vi "Build Header Frame.vi"(8 "error in (no error)":errorcluster, 9 "system info in":refnum<class "PMU System Info.lvclass">) -> (0 "error out":errorcluster, 1 "system info out":refnum<class "PMU System Info.lvclass">, 3 "header frame":string)   [LabVIEW 2013, in "NI_EP_PMU.lvlib"]
doc: "Builds a header frame as defined in IEEE Std C37.118.2-2011."
uses:
  <vilib>/addons/Electrical Power/PMU/NI_EP_PMU.lvlib
  <vilib>/addons/Electrical Power/PMU/Common/Classes/PMU System Info/PMU System Info.lvclass
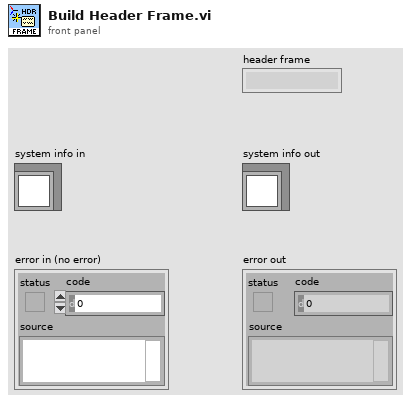
[diagram p1: front panel]
types:
  T1 = typedef "NI_EP_PMU.lvlib/pmu_CFG for Data Frame.ctl" = enum8{"CFG-2", "CFG-3"}
  T2 = typedef "NI_EP_PMU.lvlib/pmu_CFG Class.ctl" = cluster{"station name":string, "PMU ID":u16, "time base":u32, "nominal frequency":enum16{"50 Hz", "60 Hz"}, "reporting rate":i16, "phasor number":u16, "analog number":u16, "digital number":u16, "channel names":string[], "phasor units":u32[], "analog units":u32[], "digital units":u32[], "data format":u16, "number of PMUs":u16}
  T3 = typedef "NI_EP_PMU.lvlib/pmu_CFG-3 Class.ctl" = cluster{"station name":string, "PMU ID":u16, "global PMU ID":u64, "time base":u32, "nominal frequency":enum16{"50 Hz", "60 Hz"}, "reporting rate":i16, "phasor number":u16, "analog number":u16, "digital number":u16, "channel names":string[], "phasor scale first 4 bytes":u32[], "phasor scale factors":sgl[], "phasor angle offsets [rad]":sgl[], "analog scale factors":sgl[], "analog magnitude offsets":sgl[], "digital units":u32[], "data format":u16, "number of PMUs":u16}
  T4 = typedef "LVDateTimeRec.ctl" = cluster{"fractional second":dbl, "second":i32, "minute":i32, "hour":i32, "day of month":i32, "month":i32, "year":i32, "day of week":i32, "day of year":i32, "DST":i32}
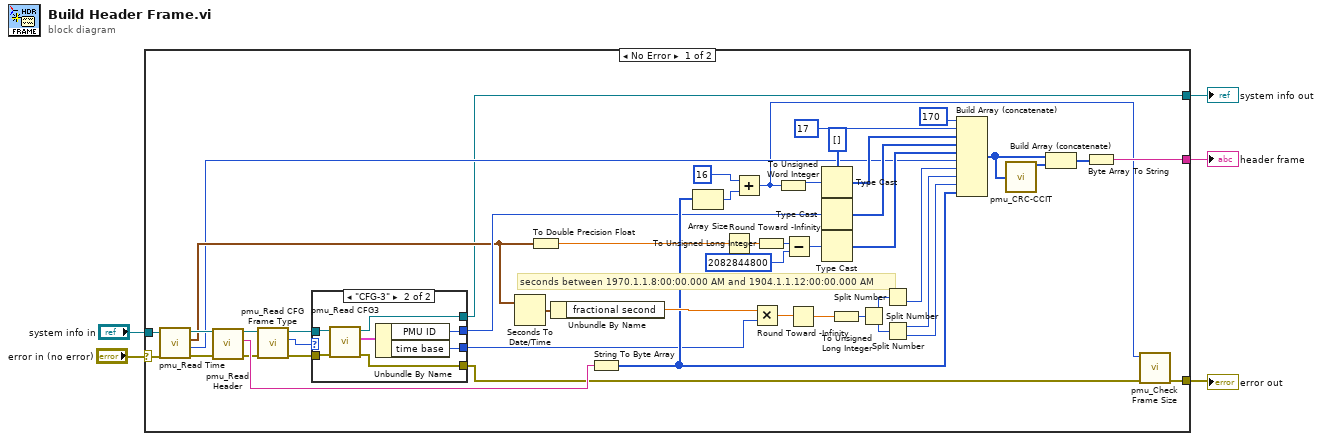
[diagram p0: block diagram]
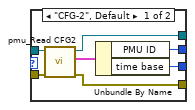
[diagram p2: hidden frame]
diagram:
  n1 = case shown="No Error" "error in (no error)" {
    selector: "error in (no error)" -> [w22 w67]
    tunnel: [w52 _] -> w5
    tunnel: [w17 w67] -> w4
    tunnel: "system info in" -> [w23 w68]
    tunnel: [w11 w68] -> w1
    frame No Error {
      w36 = u8[] [] ("appended array")
      # "seconds between 1970.1.1.8:00:00.000 AM and 1904.1.1.12:00:00.000 AM"
      n2 = call <vilib>:"pmu_Read Time.vi"("error in (no error)"=w22, "system info in"=w23) -> ("error out"=w20:errorcluster, "time quality"=w18:u8, "time stamp"=w19:timestamp, "system info out"=w21:refnum<class "PMU System Info.lvclass">)  [unwired: 6 in]
      n3 = call <vilib>:"pmu_Read Header.vi"("error in (no error)"=w20, "system info in"=w21) -> ("error out"=w15:errorcluster, "header"=w51:string, "system info out"=w16:refnum<class "PMU System Info.lvclass">)  [unwired: 7 in]
      n4 = call <vilib>:"pmu_Read CFG Frame Type.vi"("error in (no error)"=w15, "system info in"=w16) -> ("error out"=w13:errorcluster, "configuration frame option"=w12:T1, "system info out"=w14:refnum<class "PMU System Info.lvclass">)  [unwired: 7 in]
      n5 = case shown="\"CFG-3\"" w12 {
        tunnel: [w58 w61] -> w30
        tunnel: [w57 w60] -> w29
        tunnel: w14 -> [w56 w66]
        tunnel: w13 -> [w55 w65]
        tunnel: [w54 w64] -> w11
        tunnel: [w53 w63] -> w10
        frame "CFG-2", Default {
          n6 = call <vilib>:"pmu_Read CFG2.vi"("error in (no error)"=w55, "system info in"=w56) -> ("error out"=w53:errorcluster, "CFG-2"=w59:T2, "system info out"=w54:refnum<class "PMU System Info.lvclass">)  [unwired: 7 in]
          n7 = Unbundle By Name(w59) -> ("PMU ID"=w58:u16, "time base"=w57:u32)
        }
        frame "CFG-3" {
          n8 = call <vilib>:"pmu_Read CFG3.vi"("error in (no error)"=w65, "system info in"=w66) -> ("error out"=w63:errorcluster, "CFG-3"=w62:T3, "system info out"=w64:refnum<class "PMU System Info.lvclass">)  [unwired: 7 in]
          n9 = Unbundle By Name(w62) -> ("PMU ID"=w61:u16, "time base"=w60:u32)
        }
      }
      n10 = Seconds To Date/Time(time stamp (now)=w19) -> (date time rec=w34:T4)  [unwired: 1 in]
      n11 = To Double Precision Float(number=w19) -> (double precision float=w27:dbl)
      n12 = Unbundle By Name(w34) -> ("fractional second"=w32:dbl)
      n13 = String To Byte Array(string=w51) -> (unsigned byte array=w31:u8[])
      n14 = Array Size(array=w31) -> (size(s)=w9:i32)
      n15 = Round Toward -Infinity(1:w27) -> (0:w26:dbl)
      n16 = Add(x=16 ("y"), y=w9) -> (x+y=w7:i32)
      n17 = Multiply(x=w32, y=w29) -> (x*y=w25:dbl)
      n18 = To Unsigned Long Integer(number=w26) -> (unsigned 32bit integer=w33:u32)
      n19 = To Unsigned Word Integer(number=w7) -> (unsigned 16bit integer=w8:u16)
      n20 = Subtract(x=w33, y=u32 2082844800 ("unsigned 32bit integer")) -> (x-y=w38:u32)
      n21 = Round Toward -Infinity(1:w25) -> (0:w24:dbl)
      n22 = Type Cast(type=w36, x=w8) -> (*(type *) &x=w40:u8[])
      n23 = Type Cast(type=w36, x=w30) -> (*(type *) &x=w39:u8[])
      n24 = Type Cast(type=w36, x=w38) -> (*(type *) &x=w37:u8[])
      n25 = To Unsigned Long Integer(number=w24) -> (unsigned 32bit integer=w35:u32)
      n26 = Split Number(x=w35) -> (hi(x)=w46:u16, lo(x)=w47:u16)
      n27 = Split Number(x=w46) -> (lo(x)=w45:u8)  [unwired: 1 out]
      n28 = Split Number(x=w47) -> (hi(x)=w44:u8, lo(x)=w43:u8)
      n29 = Build Array (concatenate)(u8 170 ("element"), u8 17 ("element"), w40, w39, w37, w18, w45, w44, w43, w31) -> (w42:u8[])
      n30 = call <vilib>:"pmu_CRC-CCIT.vi"("byte array"=w42) -> ("CRCbytes"=w41:u8[])  [unwired: 13 in, 1 out]
      n31 = Build Array (concatenate)(w42, w41) -> (w6:u8[])
      n32 = Byte Array To String(unsigned byte array=w6) -> (string=w52:string)
      n33 = call <vilib>:"pmu_Check Frame Size.vi"("error in (no error)"=w10, "frame size"=w7) -> ("error out"=w17:errorcluster)  [unwired: 9 in]
    }
    frame Error {
    }
  }
  "header frame" <- w5
  "system info out" <- w1
  "error out" <- w4
